vi "FPGA Main R5 One Loop AB JC KV.vi"() -> ()   [LabVIEW 2018]
uses:
  Type Defs/Control Mode.ctl
  <vilib>/rvi/FXPMathLib/FxpSinAndCos/subVIs/nifxpmath_SinAndCos_SimConfig.ctl
  <vilib>/rvi/Emulation/niFpgaGetClockAttributes.vi
  <vilib>/rvi/Emulation/niFpgaSctlEmulationGetInTimedLoop.vi
  <vilib>/rvi/Emulation/niFpgaEmulationReportErrorSimple.vi
  <vilib>/rvi/Emulation/niFpgaProcessEmulError.vi
  <vilib>/rvi/eio/common/nirviEmuTemplateMethod_errors.vi
  <vilib>/rvi/interface/RandomDataEmulation/niFpgaRandomDataHandleErrors.vi
  <vilib>/rvi/Emulation/niFpgaCriticalErrorInLSC.vi
  <vilib>/rvi/FXPMathLib/FxpSinAndCos/simVIs/DllFxpSinAndCosTemp_sub.vi
  <vilib>/rvi/Analysis/control/PID/SubVIs/niFpgaPID_PIWrapper.vi
  <vilib>/eio/EIONode/EIONode.xnode
  <vilib>/rvi/DataTransferAndStorage/Container/XNode/niFpgaContainer.xnode
  <vilib>/rvi/interface/RandomDataEmulation/nirviRandomDataFpgaReadWriteTemplate.vi
  <vilib>/rvi/FXPMathLib/FxpSinAndCos/XNode/nifxpmath_SinAndCos.xnode
panel:
  out "Capacitance\nProbe (V)":u16
  out "Coil Back \nEMF (V)":u16
  in  "VC Command (V)":u16
  in  "Control Mode":T1=enum."Velocity"
  out "Current Mode":T1=enum."Velocity"
  out "Measuring?":bool
  in  "FFWD/PID":bool
  in  "Amplifier \nOn/Off":bool
  out "Array Index":i32
  out "PID Error (V)":sgl
  out "Output (V)":u16
  in  "Output Limits":cluster{"Vmax":sgl, "Vmin":sgl}
  in  "PID Gains":cluster{"Kp":sgl, "Ki":sgl}
  in  "Loop \nRate (uSec)":u32
  # "Sensors"
  # "Loop Rates"
  # "Controls"
  # "PID Settings"
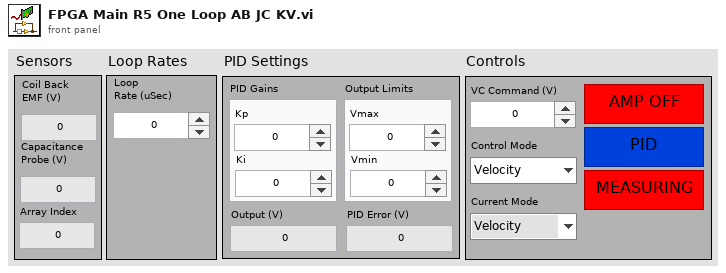
[diagram p1: front panel]
types:
  T1 = typedef "Control Mode.ctl" = enum16{"Start Velocity", "Velocity", "End Velocity", "Displacement", "Manual"}
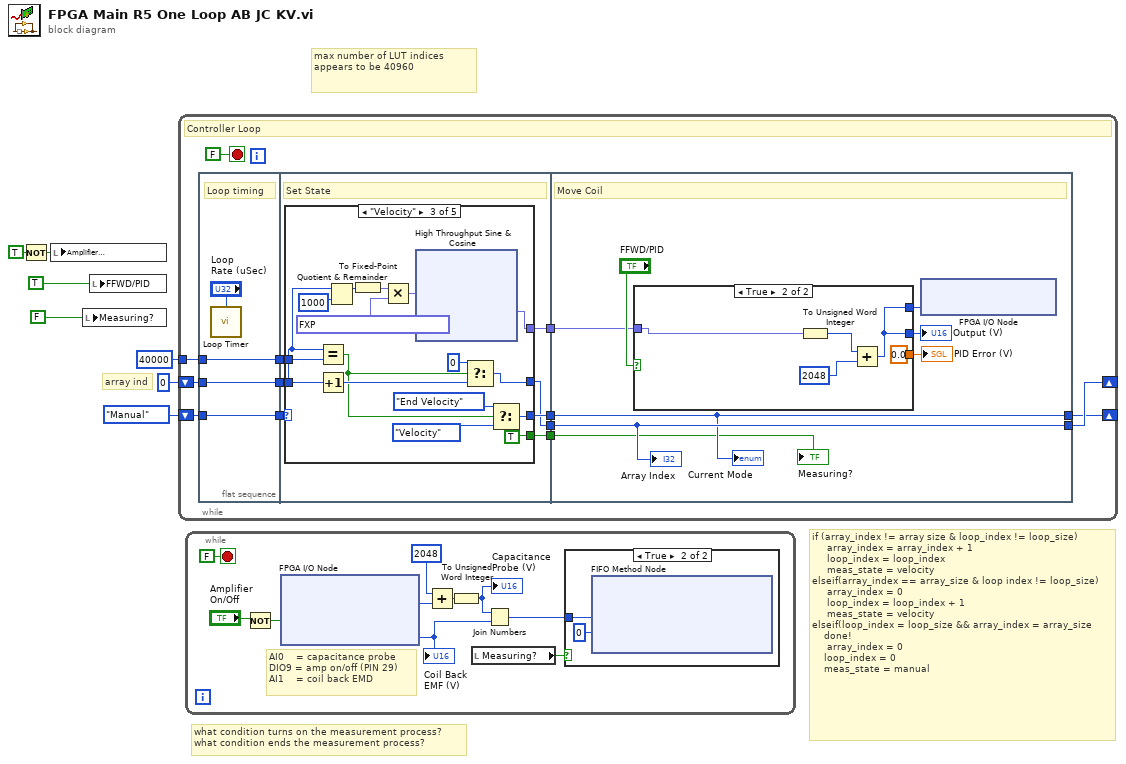
[diagram p0: block diagram]
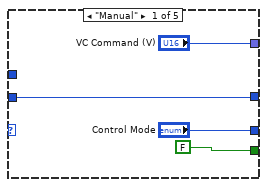
[diagram p3: hidden frame]
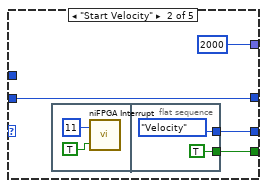
[diagram p4: hidden frame]
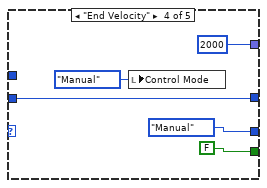
[diagram p5: hidden frame]
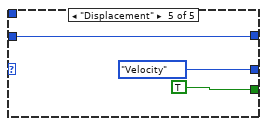
[diagram p6: hidden frame]
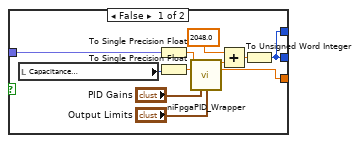
[diagram p7: hidden frame]
diagram:
  # "max number of LUT indices appears to be 40960"
  # "what condition turns on the measurement process?\nwhat condition ends the measurement process?"
  # "if (array_index != array size & loop_index != loop_size)\n     array_index = array_index + 1\n     loop_index = loop_index\n     meas_state = velocity\nelseif(array_index == array_size & loop index != loop_size)\n     array_index = 0\n     loop_index = loop_index + 1\n     meas_state = velocity\nelseif(loop_index = loop_size && array_index = array_size\n    done!\n     array_index = 0\n    loop_index = 0\n    meas_state = manual"
  # "array ind"
  n1 = Not(x=TRUE) -> (.not. x?=w4:bool)
  n2 = local write "Amplifier \nOn/Off"(w4) -> ()
  n3 = local write "Measuring?"(FALSE) -> ()
  n4 = local write "FFWD/PID"(TRUE) -> ()
  n5 = while {
    shift-right: [w10] -> _
    shift-left: 0 ("index") -> [w19]
    shift-right: [w9] -> _
    shift-left: Control_Mode."Manual" ("Control Mode") -> [w15]
    tunnel: 40000 ("index") -> [w17]
    stop <- FALSE stop-if-true
    # "Controller Loop"
    n6 = flat-sequence {
      tunnel: w19 -> [w23]
      tunnel: [w23] -> w18
      tunnel: w17 -> [w22]
      tunnel: [w22] -> w16
      tunnel: w15 -> [w21]
      tunnel: [w21] -> w14
      tunnel: w18 -> [w31]
      tunnel: w16 -> [w30]
      tunnel: w14 -> [w29]
      tunnel: [w28] -> w13
      tunnel: [w27] -> w12
      tunnel: [w26] -> w11
      tunnel: [w25] -> w8
      tunnel: [w105] -> w10
      tunnel: [w104] -> w9
      tunnel: w8 -> [w103]
      tunnel: w11 -> [w105]
      tunnel: w12 -> [w104]
      tunnel: w13 -> [w98]
      frame #0 {
        # "Loop timing"
        n7 = call "Loop Timer"("Count(uSec)"="Loop \nRate (uSec)") -> ()  [unwired: 1 out]
      }
      frame #1 {
        # "Set State"
        n8 = case shown="\"Velocity\"" w29 {
          tunnel: ["VC Command (V)" u16 2000 ("data out") w47 u16 2000 ("data out") _] -> w28
          tunnel: w31 -> [w33 w38 w50 w94 w97]
          tunnel: [w33 w38 w55 w94 w97] -> w26
          tunnel: ["Control Mode" w39 w57 Control_Mode."Manual" ("Control Mode") Control_Mode."Velocity" ("Control Mode")] -> w27
          tunnel: w30 -> [_ _ w52 _ _]
          tunnel: [FALSE w37 TRUE FALSE TRUE] -> w25
          frame "Manual" {
          }
          frame "Start Velocity" {
            n9 = flat-sequence {
              tunnel: [Control_Mode."Velocity" ("Control Mode")] -> w39
              tunnel: [TRUE] -> w37
              frame #0 {
                n10 = call <vilib>:"niFPGA Interrupt.vi"("Wait Until Cleared (F)"=TRUE, "IRQ Number (0)"=u8 11) -> ()  [unwired: 1 in]
              }
              frame #1 {
              }
            }
          }
          frame "Velocity" {
            n11 = Equal?(x=w50, y=w52) -> (x = y?=w53:bool)
            n12 = Increment(x=w50) -> (x+1=w56:i32)
            n13 = Quotient & Remainder(x=w50, y=1000) -> (x-y*floor(x/y)=w45:i32)  [unwired: 1 out]
            n14 = To Fixed-Point(number=w45) -> (fixed-point=w44:fxp<+/-,16,12>)  [unwired: 1 in]
            n15 = Multiply(x=w44, y=fxp<+,16,-8> 0.001999974250793457) -> (x*y=w46:fxp<+/-,32,4>)
            n16 = xnode "High Throughput Sine & Cosine"("x (pi)"=w46) -> ("sin(x)"=w47:fxp<+/-,16,2>)  [unwired: 1 out]
            n17 = Select(t=0 ("index"), s=w53, f=w56) -> (s? t:f=w55:i32)
            n18 = Select(t=Control_Mode."End Velocity" ("Control Mode"), s=w53, f=Control_Mode."Velocity" ("Control Mode")) -> (s? t:f=w57:T1)
          }
          frame "End Velocity" {
            n19 = local write "Control Mode"(Control_Mode."Manual" ("Control Mode")) -> ()
          }
          frame "Displacement" {
          }
        }
      }
      frame #2 {
        # "Move Coil"
        n20 = case shown="True" "FFWD/PID" {
          tunnel: w98 -> [w115 w120]
          tunnel: [w106 w117] -> w99
          tunnel: [w109 sgl 0.0 ("error")] -> w100
          tunnel: [w106 w117] -> w102
          frame False {
            n21 = local read "Capacitance\nProbe (V)"() -> (w113:u16)
            n22 = To Single Precision Float(number=w115) -> (single precision float=w114:sgl)
            n23 = To Single Precision Float(number=w113) -> (single precision float=w116:sgl)
            n24 = call-poly <vilib>:"niFpgaPID_Wrapper.vi"("setpoint"=w114, "process variable"=w116, "gains"="PID Gains", "output range"="Output Limits") -> ("output"=w108:sgl, "error"=w109:sgl)  [unwired: 9 in, 1 out]
            n25 = Add(x=sgl 2048.0, y=w108) -> (x+y=w110:sgl)
            n26 = To Unsigned Word Integer(number=w110) -> (unsigned 16bit integer=w106:u16)
          }
          frame True {
            n27 = To Unsigned Word Integer(number=w120) -> (unsigned 16bit integer=w118:u16)
            n28 = Add(x=w118, y=i16 2048) -> (x+y=w117:u16)
          }
        }
        "Output (V)" <- w99
        "PID Error (V)" <- w100
        n29 = xnode "FPGA I/O Node"("ConnectorA/AO1"=w102) -> ()  [unwired: 1 in, 1 out]
        "Measuring?" <- w103
        "Array Index" <- w105
        "Current Mode" <- w104
      }
    }
  }
  n30 = while {
    stop <- FALSE stop-if-true
    # "AI0    = capacitance probe\nDIO9 = amp on/off (PIN 29)\nAI1    = coil back EMD"
    n31 = Not(x="Amplifier \nOn/Off") -> (.not. x?=w128:bool)
    n32 = xnode "FPGA I/O Node"("ConnectorA/DIO9"=w128) -> ("ConnectorC/AI0"=w130:i16, "ConnectorA/AI1"=w122:u16)  [unwired: 3 in, 3 out]
    "Coil Back \nEMF (V)" <- w122
    n33 = Add(x=i16 2048, y=w130) -> (x+y=w131:i16)
    n34 = To Unsigned Word Integer(number=w131) -> (unsigned 16bit integer=w123:u16)
    "Capacitance\nProbe (V)" <- w123
    n35 = local read "Measuring?"() -> (w125:bool)
    n36 = Join Numbers(hi=w123, lo=w122) -> ((hi.lo)=w129:u32)
    n37 = case shown="True" w125 {
      tunnel: w129 -> [_ w133]
      frame False {
      }
      frame True {
        n38 = xnode ("FIFO Method Node")("Element"=w133, "Timeout"=0) -> ()  [unwired: 1 in, 2 out]
      }
    }
  }
